vi "Stop Work.vi"(6 "Controller name":string, 8 "error in (no error)":errorcluster, 9 "Reply":bool=TRUE, 10 "Reply to":refnum<class "Stop Response Msg.lvclass">, 11 "Measure Object in":refnum<class "Pulse Recorder Actor.lvclass">) -> (0 "error out":errorcluster, 3 "Measure Object out":refnum<class "Pulse Recorder Actor.lvclass">)   [LabVIEW 2021, in "Pulse Recorder Actor.lvclass"]
uses:
  Pulse Recorder Actor.lvclass
  Controllers/Process Controller Messages/Stop Response Msg/Stop Response Msg.lvclass
  Instrument Actor/Instrument Actor.lvclass
  Pulse Recorder Actor.lvclass/Pulse Recorder Actor.ctl
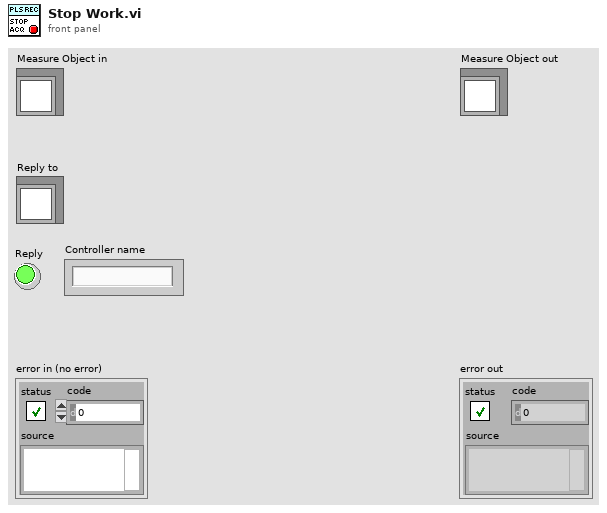
[diagram p1: front panel]
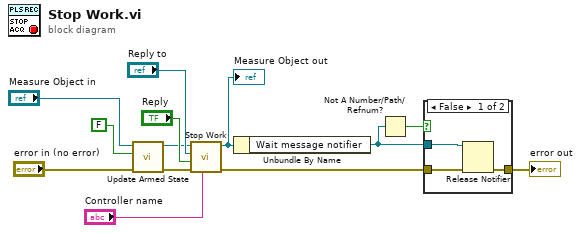
[diagram p0: block diagram]
diagram:
  n1 = call-dynamic "Update Armed State.vi"("error in (no error)"="error in (no error)", "Armed"=FALSE, "Pulse Recorder in"="Measure Object in") -> ("error out"=w9:errorcluster, "Pulse Recorder out"=w6:refnum<class "Pulse Recorder Actor.lvclass">)  [unwired: 7 in]
  n2 = call-parent "Stop Work.vi"("Controller name"="Controller name", "error in (no error)"=w9, "Reply"="Reply", "Reply to"="Reply to", "Measure Object in"=w6) -> ("error out"=w2:errorcluster, "Measure Object out"=w3:refnum<class "Pulse Recorder Actor.lvclass">)  [unwired: 5 in]
  "Measure Object out" <- w3
  n3 = Unbundle By Name(w3) -> ("Wait message notifier"=w5:refnum<notifier>)
  n4 = Not A Number/Path/Refnum?(number/path/refnum=w5) -> (NaN/Path/Refnum?=w4:bool)
  n5 = case shown="False" w4 {
    tunnel: w2 -> [w16 w17]
    tunnel: [w15 w17] -> w1
    tunnel: w5 -> [w14 _]
    frame False {
      n6 = Release Notifier(notifier=w14, error in (no error)=w16) -> (error out=w15:errorcluster)  [unwired: 1 in, 2 out]
    }
    frame True {
    }
  }
  "error out" <- w1
